vi "Set EDS File Path.vi"(8 "error in":errorcluster, 10 "EDS File Path":path, 11 "reference in":refnum<class "Electronic Datasheet.lvclass">) -> (0 "error out":errorcluster, 3 "reference out":refnum<class "Electronic Datasheet.lvclass">)   [LabVIEW 2024, in "Electronic Datasheet.lvlib" / "Electronic Datasheet.lvclass"]
uses:
  Electronic Datasheet.lvclass
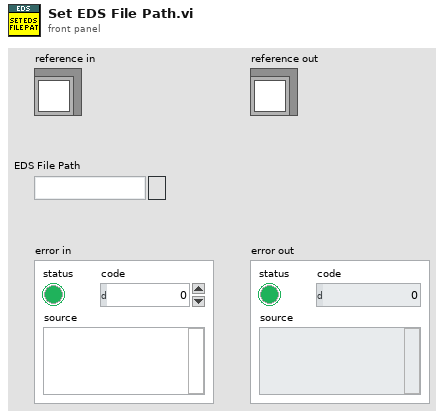
[diagram p1: front panel]
types:
  T1 = typedef "Electronic Datasheet.lvlib/Electronic Datasheet.lvclass/ObjectAttributes.ctl" = cluster{"EDS File Path":path, "Object Dict":refnum<class "Dictionary.lvclass">, "Sorted Object Dict":refnum<class "Sorted Object Dictionary.lvclass">, "Device Info":refnum<class "Device Info.lvclass">, "File Info":refnum<class "File Info.lvclass">}
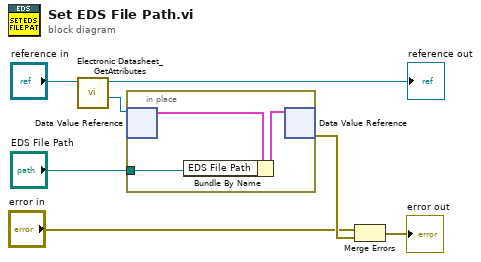
[diagram p0: block diagram]
diagram:
  n1 = call "Electronic Datasheet_GetAttributes.vi"("reference in"="reference in") -> ("DataRef"=w4:refnum<data-value>, "reference out"=→"reference out":refnum<class "Electronic Datasheet.lvclass">)  [unwired: 7 in, 2 out]
  n2 = in-place {
    in-place-border: "EDS File Path" -> [w8]
    n3 = in-place-dvr #1(w4) -> (w10:T1)  [unwired: 1 out]
    n4 = Bundle By Name(cluster=w10, "EDS File Path"=w8) -> (w9:T1)
    n5 = in-place-dvr #1(w9) -> (w5:errorcluster)  [unwired: 1 out]
  }
  n6 = Merge Errors("error in", w5) -> (→"error out":errorcluster)
